vi "Check-filename.vi"(11 "Filename":string) -> (2 "Filename (Evaluated)":string)   [LabVIEW 2018]
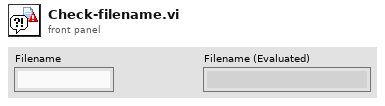
[diagram p1: front panel]
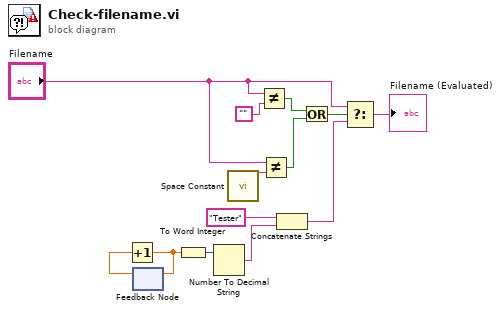
[diagram p0: block diagram]
diagram:
  n1 = feedback #1() -> (w6:dbl)  [unwired: 1 in]
  n2 = Increment(x=w6) -> (x+1=w3:dbl)
  n3 = feedback-in #1(w3) -> ()
  n4 = To Word Integer(number=w3) -> (16bit integer=w4:i16)
  n5 = Number To Decimal String(number=w4) -> (decimal integer string=w5:string)  [unwired: 1 in]
  n6 = call <vilib>:"Space Constant.vi"() -> ("String"=w10:string)
  n7 = Not Equal?(x="Filename", y="") -> (x != y?=w11:bool)
  n8 = Not Equal?(x="Filename", y=w10) -> (x != y?=w9:bool)
  n9 = Concatenate Strings("Tester" ("string"), w5) -> (w2:string)
  n10 = Or(x=w11, y=w9) -> (x .or. y?=w8:bool)
  n11 = Select(t="Filename", s=w8, f=w2) -> (s? t:f=→"Filename (Evaluated)":string)
